vi "Create_Results_Row.vi"() -> (0 "row splitting":string[][](array[string]), 1 "Values to Keep in Dup rows":bool[](array[boolean]), 2 "Channel Values":string[](array[string]), 3 "Channel Names":string[](array[string]))   [LabVIEW 2015]
uses:
  Globals/Meas_global.vi
  Globals/Trav_pos_global.vi
  Globals/Dynamic_call_global.ph.vi
  Globals/Extra_Commands_Global.vi
  Globals/LDA_meas_global_1.vi
  Acquisition/PWA/PWAtasksGLOBAL.vi
panel:
  out "ScrollableArray":T1(array[cluster])
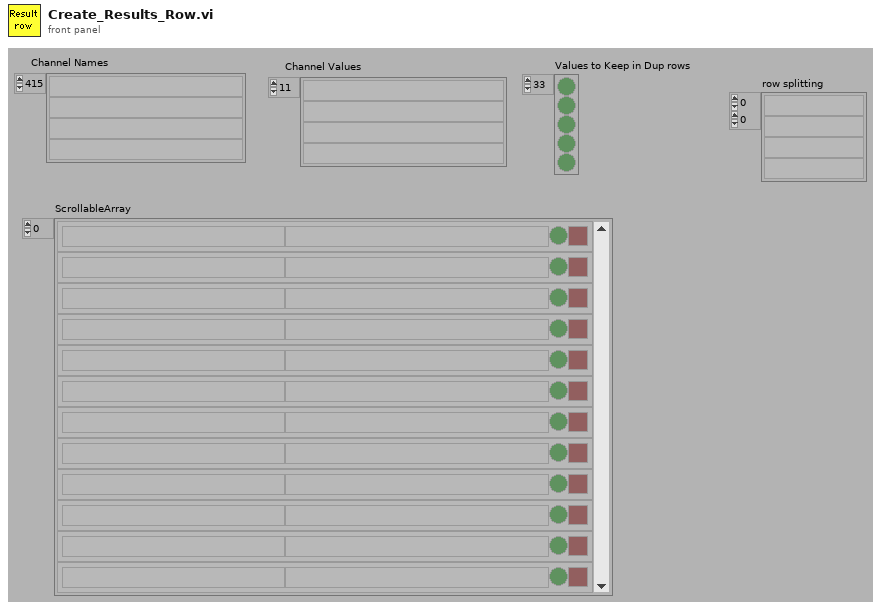
[diagram p1: front panel]
types:
  T1 = cluster{"Input Element":string, "name":string, bool, bool}[]
  T2 = typedef "Analysis_info_cluster.ctl" = cluster{"Colour":u32, "Inst type":T3, "Inst name":string, "Symbol":string, "Code name":string, "Extra Info":string, "Inst Array":T4, "Extra Titles":string[], "Extra Values":string[], "U":dbl, "u^2":dbl, "u^3":dbl, "u^4":dbl, "Skew_u":dbl, "Kurt_u":dbl, "Sd Error in Mean":dbl, "% u'/U":dbl, "X":dbl, "Y":dbl, "Z":dbl, "Timescale integral to 25%":dbl, "Sd Error in Variance":dbl, "Calib File":path, "Calib Constants":dbl[], "Output Position":bool, "Full Stats":bool, "Av Sampling Rate":dbl, "Av No of Samples":dbl, "Total Meas Time (s)":dbl, "ADAM Ch Name":string, "Max value":dbl, "Min value":dbl}
  T3 = typedef "Inst_type.ctl" = enum16{"Propeller anemometer", "Raw voltage", "Pressure Transducer", "Pitot-static tube", "Preston tube", "Hot wire", "Cross wire 1", "Cross wire 2", "Generic Linear", "Generic Polynomial", "Generic BackPoly", "Fast FID", "Thermocouple", "Cold wire", "Pulsed Wire", "LDA Vel", "LDA Tran time", "LDA Arr time", "Microphone"}
  T4 = typedef "Instrument_Array.ctl" = enum16{"PWA", "LDA", "Analogue"}
  T5 = typedef "Post_Process.ctl" = enum16{"Take New Data", "Post Process Raw Data File"}
  T6 = typedef "PWA_Data.ctl" = enum16{"No PWA Data", "One Ch PWA"}
  T7 = typedef "Correlation_cluster1.ctl" = cluster{"U inst":string, "uw":dbl, "u^2w":dbl, "uw^2":dbl, "uw/u'w'":dbl, "W inst":string, "uw^3":dbl, "u^3w":dbl, "u^2w^2":dbl, "Index U":i32, "Index W":i32}
  T8 = typedef "Traverse_cluster.ctl" = cluster{"Start X":sgl, "Start Y":sgl, "Start Z":sgl, "End X":sgl, "End Y":sgl, "End Z":sgl, "No. of pts.":i32, "Spacing":T9, "Filename":path, "Tunnel Speed":dbl, "Averaging time (min)":dbl, "Extra Commands":string, "Carrier_1 Q (l/min)":dbl, "Carrier_2 Q (l/min)":dbl, "Trace Gas Concentration (%)":dbl, "Specific Arguments":string, "Comments":string, "Row No":i32, "Row Type Selector":T10, "Completion time":string, "Row Duration (mins)":dbl, "No. of Valid pts.":i32, "Meas Setup File":string}
  T9 = typedef "Spacing.ctl" = enum16{"Linear", "Log", "Gauss", "Specified", "N/A"}
  T10 = typedef "Multi_run_mode.ctl" = enum16{"Move Traverse Only", "Set Tunnel Speed Only", "Set Source Only", "Set Measurement Conditions", "Single Measurement", "Vertical Profile", "Lateral Profile", "Longitudinal Profile", "Explore Volume", "Multi-Axis Profile", "Auto Calibrate", "Meas Fast FID Bkgnd", "Check Beam Power", "Scanning Valve Measurement", "Run VI Named:", "Set ADAM Ch", "Wait (minutes)", "Send Message", "Synchronize With:", "Fall Back to this Row", "Turn Off Row Repeating", "Blank Row", "Traverse 3D Volume"}
  T11 = cluster{"Input Element":string, "name":string, bool, bool}
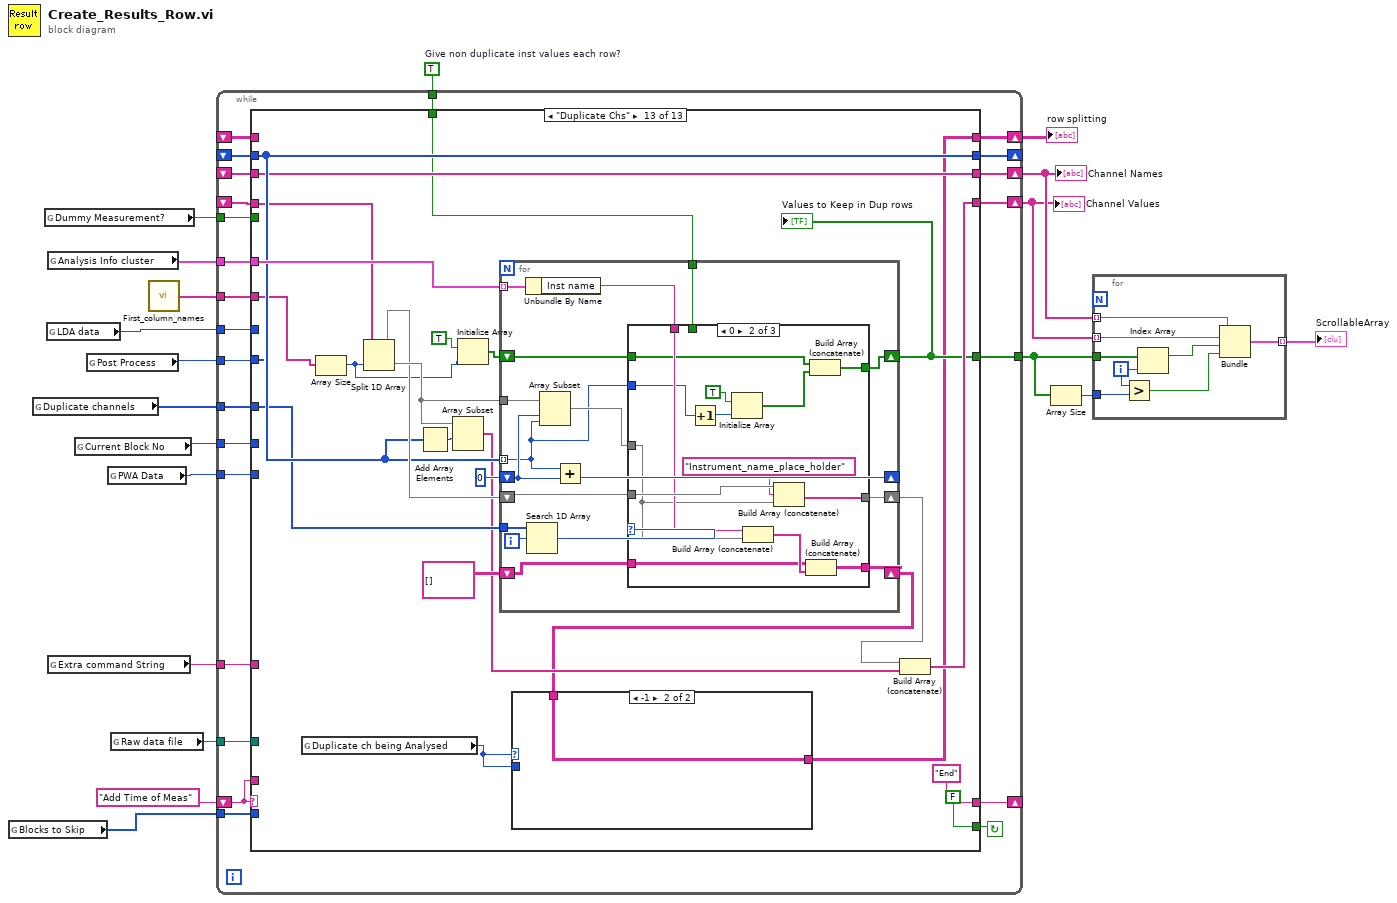
[diagram p0: block diagram]
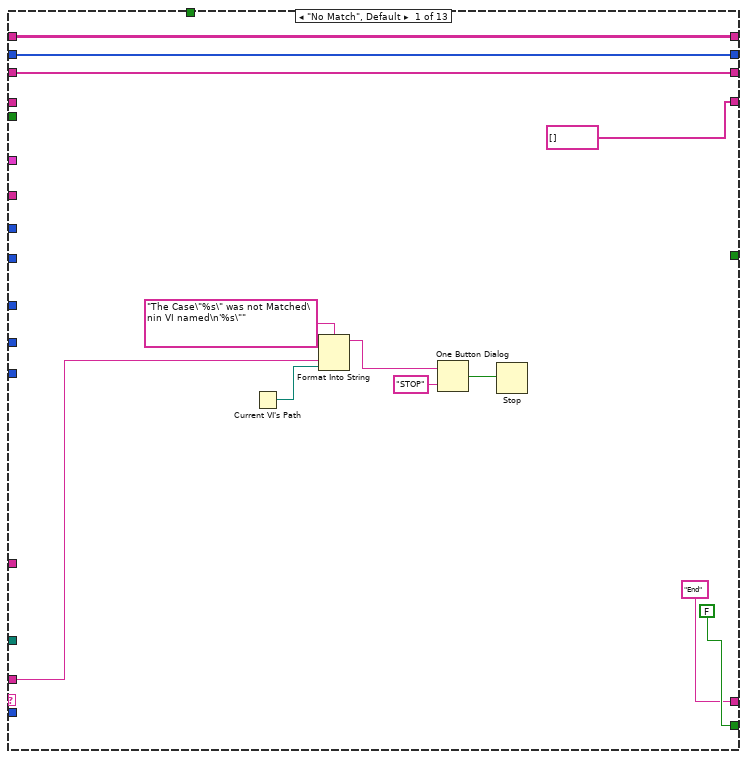
[diagram p2: hidden frame]
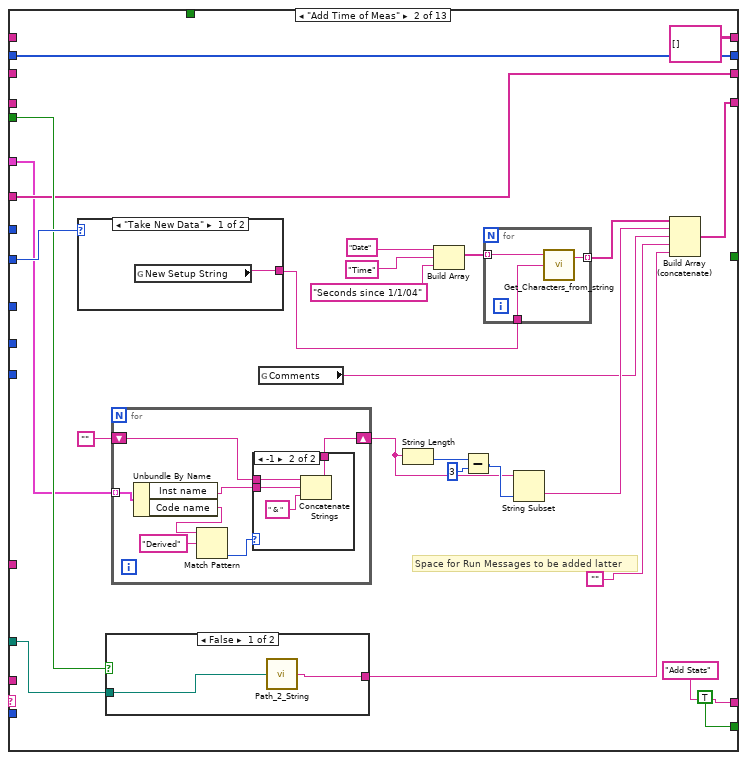
[diagram p3: hidden frame]
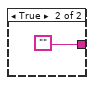
[diagram p4: hidden frame]
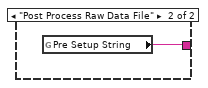
[diagram p6: hidden frame]
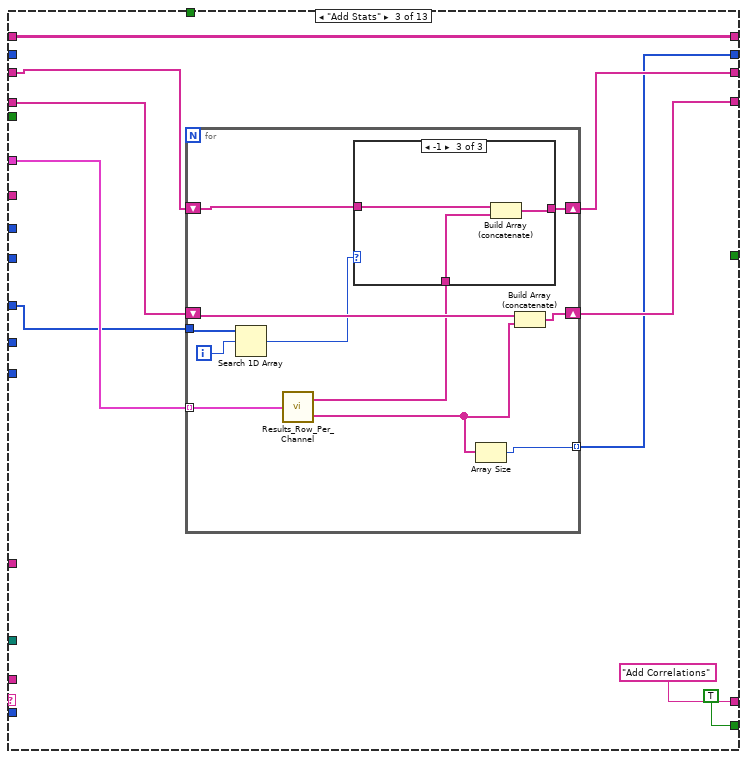
[diagram p7: hidden frame]
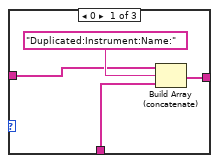
[diagram p8: hidden frame]
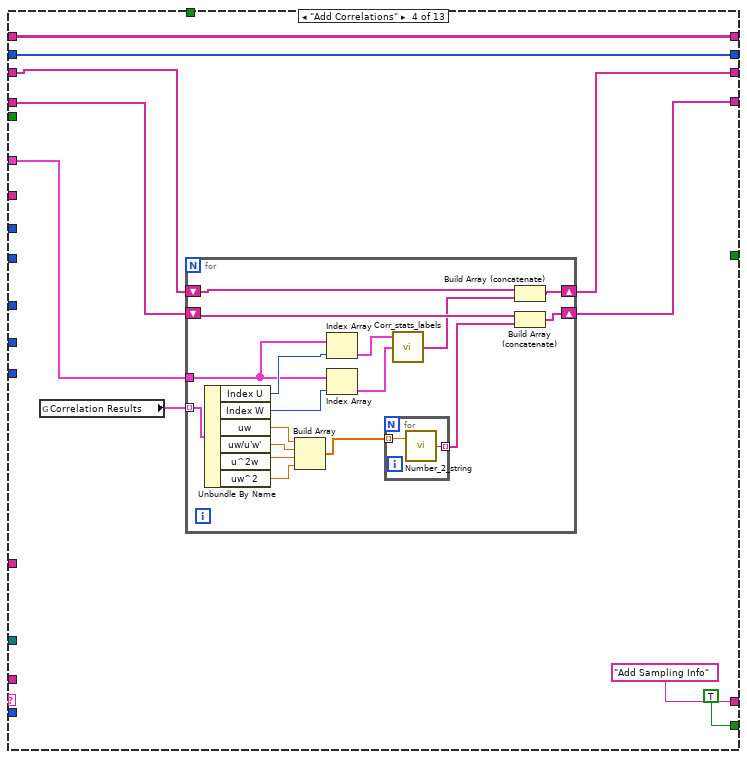
[diagram p10: hidden frame]
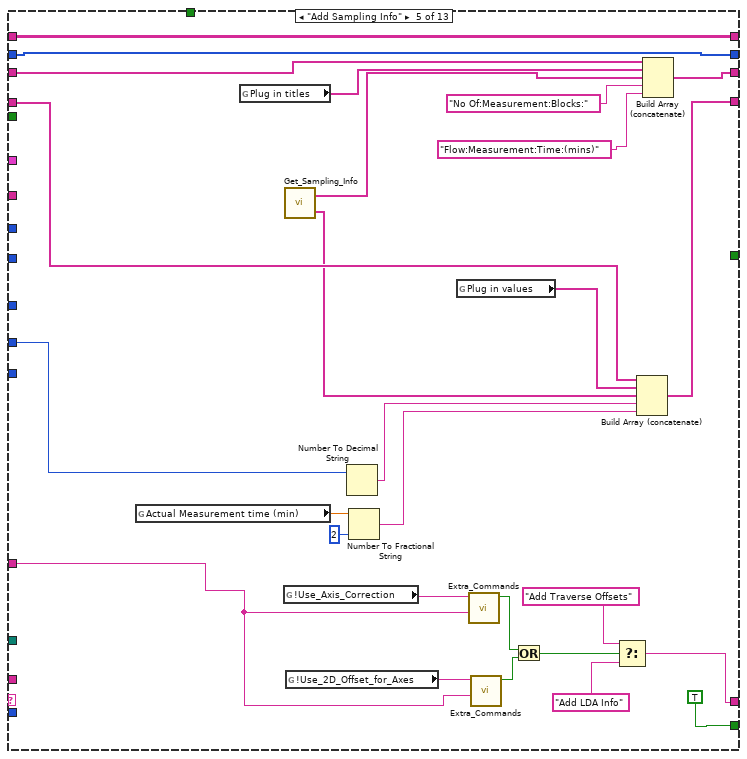
[diagram p11: hidden frame]
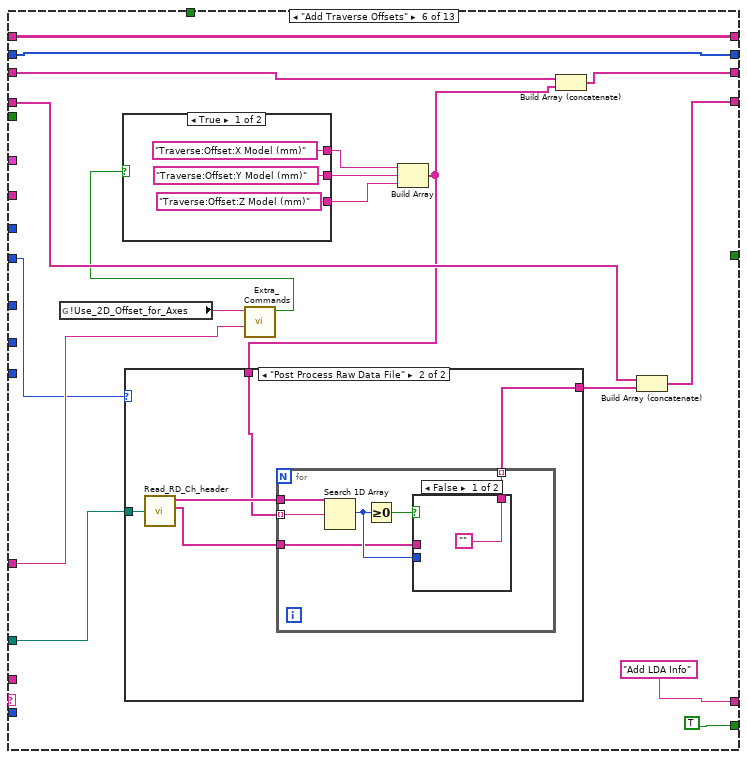
[diagram p12: hidden frame]
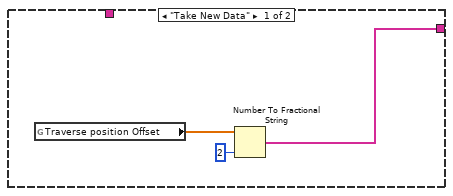
[diagram p13: hidden frame]
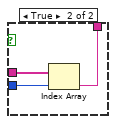
[diagram p14: hidden frame]
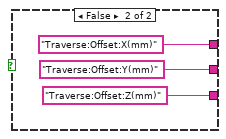
[diagram p15: hidden frame]
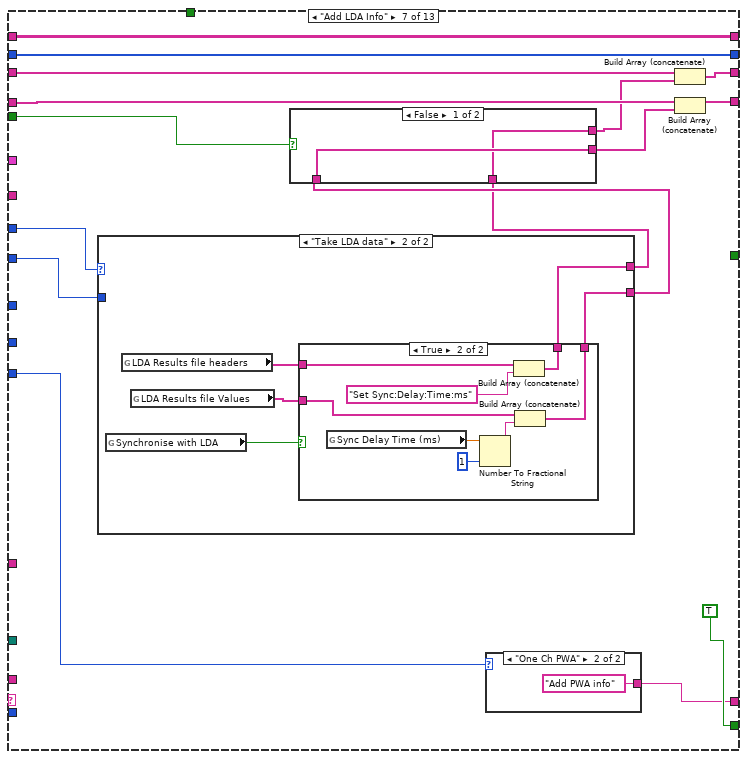
[diagram p16: hidden frame]
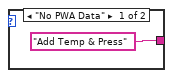
[diagram p17: hidden frame]
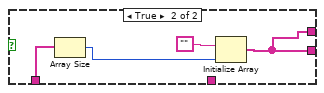
[diagram p18: hidden frame]
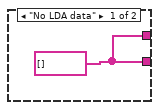
[diagram p19: hidden frame]
diagram:
  w1 = TRUE  # Give non duplicate inst values each row?
  n1 = global read "Meas_global.vi" "Blocks to Skip"() -> (w13:i32[])
  n2 = global read "Meas_global.vi" "Duplicate channels"() -> (w10:i32[])
  n3 = global read "Trav_pos_global.vi" "Dummy Measurement?"() -> (w15:bool)
  n4 = global read "Meas_global.vi" "LDA data"() -> (w19:enum16{"No LDA data", "Take LDA data"})
  n5 = global read "Meas_global.vi" "Analysis Info cluster"() -> (w17:T2[])
  n6 = global read "Meas_global.vi" "Extra command String"() -> (w7:string)
  n7 = global read "Meas_global.vi" "Current Block No"() -> (w18:i32)
  n8 = global read "Meas_global.vi" "Post Process"() -> (w16:T5)
  n9 = global read "Meas_global.vi" "PWA Data"() -> (w12:T6)
  n10 = global read "Meas_global.vi" "Raw data file"() -> (w11:path)
  n11 = call "First_column_names.vi"() -> ("Array"=w9:string[])
  n12 = while {
    shift-left: _ -> [w36]
    shift-right: [w37] -> w5
    shift-left: "Add Time of Meas" -> [w32]
    shift-right: [w38] -> _
    tunnel: w16 -> [w40]
    tunnel: w17 -> [w41]
    tunnel: w18 -> [w42]
    tunnel: w19 -> [w43]
    tunnel: w15 -> [w35]
    shift-right: [w34] -> w6
    shift-left: _ -> [w33]
    tunnel: w13 -> [w31]
    tunnel: w12 -> [w30]
    tunnel: w11 -> [w29]
    tunnel: w10 -> [w28]
    shift-right: [w27] -> _
    shift-left: _ -> [w26]
    tunnel: w9 -> [w25]
    shift-right: [w24] -> w8
    shift-left: _ -> [w23]
    tunnel: w7 -> [w22]
    tunnel: [w21] -> w4
    tunnel: w1 -> [w20]
    stop <- w39 continue-if-true
    n13 = case shown="\"Duplicate Chs\"" w32 {
      tunnel: w41 -> [_ w57 w106 w132 _ _ _ _ _ _ _ _ w518]
      tunnel: w43 -> [_ _ _ _ _ _ w241 _ _ _ _ _ _]
      tunnel: w42 -> [_ _ _ _ w181 _ _ w280 _ _ _ _ _]
      tunnel: w40 -> [_ w64 _ _ _ w190 w236 _ w354 _ w447 w489 _]
      tunnel: [FALSE ("Processing last block?") TRUE TRUE ("Processing last block?") TRUE ("Processing last block?") TRUE TRUE TRUE ("Processing last block?") TRUE ("Processing last block?") TRUE ("Processing last block?") TRUE ("Processing last block?") TRUE ("Processing last block?") w485 FALSE ("Processing last block?")] -> w39
      tunnel: ["End" "Add Stats" "Add Correlations" ("t") "Add Sampling Info" ("t") w161 "Add LDA Info" w230 "Add Temp & Press" "Replace Run Messages" "Add Plugins" "Add Original Results filename" "Duplicate Chs" "End" ("t")] -> w38
      tunnel: [string[] [] ("initialized array") w56 w107 w136 w180 w200 w242 w281 w362 w416 w442 w494 w511] -> w37
      tunnel: w36 -> [_ _ w108 w137 w177 w199 w243 w268 w349 w402 w448 w492 w515]
      tunnel: w32 -> [w50 _ _ _ _ _ _ _ _ _ _ _ _]
      tunnel: w35 -> [_ w63 _ _ _ _ w240 _ _ w410 _ _ _]
      tunnel: [w47 w59 w109 w138 w175 w187 w233 w271 w343 w408 w438 w482 w510] -> w34
      tunnel: w33 -> [w47 _ w110 w139 w176 w188 w234 w272 w348 w408 w440 w483 w510]
      tunnel: w31 -> [_ _ _ _ _ _ _ _ _ w404 _ _ _]
      tunnel: w30 -> [_ _ _ _ _ _ w231 _ _ _ _ _ _]
      tunnel: w29 -> [_ w61 _ _ _ w189 _ _ w353 _ _ _ _]
      tunnel: w28 -> [_ _ w103 _ _ _ _ _ _ _ _ w487 w514]
      tunnel: [w46 w60 w102 w131 w172 w198 w229 w270 w345 w401 w437 w488 w517] -> w27
      tunnel: w26 -> [w46 w60 _ w131 w172 w198 w229 w270 w345 w401 w437 w488 w517]
      tunnel: w25 -> [_ w59 _ _ _ _ _ _ _ _ _ _ w516]
      tunnel: [w45 string[][] [] w101 w130 w171 w197 w228 w269 w344 w400 w436 w484 w502] -> w24
      tunnel: w23 -> [w45 _ w101 w130 w171 w197 w228 w269 w344 w400 w436 w484 _]
      tunnel: w22 -> [_ _ _ _ w160 w192 _ _ _ _ _ _ _]
      tunnel: [_ _ _ _ _ _ _ _ _ _ _ _ w504] -> w21
      tunnel: w20 -> [_ _ _ _ _ _ _ _ _ _ _ _ w503]
      frame "No Match", Default {
        n14 = Current VI's Path() -> (path=w51:path)
        n15 = Format Into String(format string="The Case\"%s\" was not Matched\nin VI named\n'%s\"" ("Format String"), w50, w51) -> (resulting string=w54:string)  [unwired: 2 in, 1 out]
        n16 = One Button Dialog(message=w54, button name ("OK")="STOP") -> (true=w52:bool)
        n17 = Stop(stop? (T)=w52) -> ()
      }
      frame "Add Time of Meas" {
        # "Space for Run Messages to be added latter"
        n18 = case shown="\"Take New Data\"" w64 {
          tunnel: [w99 w100] -> w74
          frame "Take New Data" {
            n19 = global read "Meas_global.vi" "New Setup String"() -> (w99:string)
          }
          frame "Post Process Raw Data File" {
            n20 = global read "Meas_global.vi" "Pre Setup String"() -> (w100:string)
          }
        }
        n21 = case shown="False" w63 {
          tunnel: [w82 ""] -> w72
          tunnel: w61 -> [w81 _]
          frame False {
            n22 = call "Path_2_String.vi"("Real Path"=w81) -> ("Path String"=w82:string)
          }
          frame True {
          }
        }
        n23 = for {
          shift-right: [w89] -> w67
          shift-left: "" -> [w90]
          tunnel: w57 -> [w88] mode=indexing
          n24 = Unbundle By Name(w88) -> ("Inst name"=w87:string, "Code name"=w86:string)
          n25 = Match Pattern(string=w86, regular expression="Derived") -> (offset past match=w84:i32)  [unwired: 1 in, 3 out]
          n26 = case shown="-1" w84 {
            tunnel: w90 -> [w91 w95]
            tunnel: [w91 w94] -> w89
            tunnel: w87 -> [_ w92]
            frame 0, Default {
            }
            frame -1 {
              n27 = Concatenate Strings(w95, w92, " & ") -> (w94:string)
            }
          }
        }
        n28 = global read "Meas_global.vi" "Comments"() -> (w62:string)
        n29 = String Length(string=w67) -> (length=w70:i32)
        n30 = Build Array("Date", "Time", "Seconds since 1/1/04") -> (w76:string[])
        n31 = Subtract(x=w70, y=3) -> (x-y=w68:i32)
        n32 = for {
          tunnel: w76 -> [w98] mode=indexing
          tunnel: w74 -> [w97]
          tunnel: [w96] -> w75 mode=indexing
          n33 = call "Get_Characters_from_string.vi"("Input string"=w97, "Variable name"=w98) -> ("Value"=w96:string)  [unwired: 1 in, 1 out]
        }
        n34 = String Subset(string=w67, length (rest)=w68) -> (substring=w65:string)  [unwired: 1 out]
        n35 = Build Array (concatenate)(w75, w65, w62, "", w72) -> (w56:string[])
      }
      frame "Add Stats" {
        n36 = for {
          shift-right: [w118] -> w109
          shift-left: w110 -> [w120]
          shift-right: [w121] -> w107
          shift-left: w108 -> [w119]
          tunnel: w106 -> [w117] mode=indexing
          tunnel: [w114] -> w102 mode=indexing
          tunnel: w103 -> [w112]
          i -> [w113]
          n37 = Search 1D Array(1D array=w112, element=w113) -> (index of element=w111:i32)  [unwired: 1 out]
          n38 = call "Results_Row_Per_Channel.vi"("Analysis_info_cluster"=w117) -> ("Channel Names"=w116:string[], "Channel Values"=w115:string[])
          n39 = case shown="-1" w111 {
            tunnel: w120 -> [w124 w126 w129]
            tunnel: [w122 w126 w128] -> w118
            tunnel: w116 -> [w123 _ w127]
            frame 0 {
              n40 = Build Array (concatenate)(w124, "Duplicated:Instrument:Name:", w123) -> (w122:string[])
            }
            frame 1, Default {
            }
            frame -1 {
              n41 = Build Array (concatenate)(w129, w127) -> (w128:string[])
            }
          }
          n42 = Array Size(array=w115) -> (size(s)=w114:i32)
          n43 = Build Array (concatenate)(w119, w115) -> (w121:string[])
        }
      }
      frame "Add Correlations" {
        n44 = global read "Meas_global.vi" "Correlation Results"() -> (w133:T7[])
        n45 = for {
          shift-right: [w153] -> w138
          shift-left: w139 -> [w155]
          shift-right: [w156] -> w136
          shift-left: w137 -> [w154]
          tunnel: w133 -> [w152] mode=indexing
          tunnel: w132 -> [w149]
          n46 = Unbundle By Name(w152) -> ("Index U"=w151:i32, "Index W"=w150:i32, "uw"=w145:dbl, "uw/u'w'"=w144:dbl, "u^2w"=w143:dbl, "uw^2"=w142:dbl)
          n47 = Build Array(w145, w144, w143, w142) -> (w141:dbl[])
          n48 = Index Array(array=w149, index=w151) -> (element=w148:T2)
          n49 = Index Array(array=w149, index=w150) -> (element=w147:T2)
          n50 = for {
            tunnel: w141 -> [w158] mode=indexing
            tunnel: [w157] -> w140 mode=indexing
            n51 = call "Number_2_string.vi"("number"=w158) -> ("String"=w157:string)  [unwired: 1 in]
          }
          n52 = call "Corr_stats_labels.vi"("Inst 2 Units"=w147, "Inst 1 Units"=w148) -> ("Output"=w146:string[])  [unwired: 1 in]
          n53 = Build Array (concatenate)(w155, w146) -> (w153:string[])
          n54 = Build Array (concatenate)(w154, w140) -> (w156:string[])
        }
      }
      frame "Add Sampling Info" {
        n55 = global read "Meas_global.vi" "Actual Measurement time (min)"() -> (w182:dbl)
        n56 = global read "Dynamic_call_global.ph.vi" "Plug in titles"() -> (w174:string[])
        n57 = global read "Extra_Commands_Global.vi" "!Use_Axis_Correction"() -> (w164:string)
        n58 = call "Get_Sampling_Info.vi"() -> ("Channel Values"=w169:string[], "Channel Names"=w170:string[])  [unwired: 2 in]
        n59 = global read "Extra_Commands_Global.vi" "!Use_2D_Offset_for_Axes"() -> (w165:string)
        n60 = Number To Decimal String(number=w181) -> (decimal integer string=w179:string)  [unwired: 1 out]
        n61 = Number To Fractional String(number=w182, precision (6)=i16 2) -> (F-format string=w184:string)  [unwired: 2 out]
        n62 = global read "Dynamic_call_global.ph.vi" "Plug in values"() -> (w178:string[])
        n63 = call "Extra_Commands.vi"("String to Search"=w160, "Command"=w164) -> ("Command Found"=w166:bool)  [unwired: 1 in, 4 out]
        n64 = call "Extra_Commands.vi"("String to Search"=w160, "Command"=w165) -> ("Command Found"=w167:bool)  [unwired: 1 in, 4 out]
        n65 = Or(x=w166, y=w167) -> (x .or. y?=w159:bool)
        n66 = Select(t="Add Traverse Offsets", s=w159, f="Add LDA Info") -> (s? t:f=w161:string)
        n67 = Build Array (concatenate)(w177, w178, w169, w179, w184) -> (w180:string[])
        n68 = Build Array (concatenate)(w176, w174, w170, "No Of:Measurement:Blocks:", "Flow:Measurement:Time:(mins)") -> (w175:string[])
      }
      frame "Add Traverse Offsets" {
        n69 = global read "Extra_Commands_Global.vi" "!Use_2D_Offset_for_Axes"() -> (w193:string)
        n70 = call "Extra_Commands.vi"("String to Search"=w192, "Command"=w193) -> ("Command Found"=w191:bool)  [unwired: 1 in, 4 out]
        n71 = case shown="True" w191 {
          tunnel: ["Traverse:Offset:X Model (mm)" "Traverse:Offset:X(mm)"] -> w196
          tunnel: ["Traverse:Offset:Y Model (mm)" "Traverse:Offset:Y(mm)"] -> w195
          tunnel: ["Traverse:Offset:Z Model (mm)" "Traverse:Offset:Z(mm)"] -> w194
          frame True {
          }
          frame False {
          }
        }
        n72 = Build Array(w196, w195, w194) -> (w186:string[])
        n73 = case shown="\"Post Process Raw Data File\"" w190 {
          tunnel: [w206 w207] -> w201
          tunnel: w189 -> [_ w209]
          tunnel: w186 -> [_ w208]
          frame "Take New Data" {
            n74 = global read "Trav_pos_global.vi" "Traverse position Offset"() -> (w204:sgl[])
            n75 = Number To Fractional String(number=w204, precision (6)=i16 2) -> (F-format string=w206:string[])  [unwired: 2 out]
          }
          frame "Post Process Raw Data File" {
            n76 = call "Read_RD_Ch_header.vi"("Raw data file"=w209) -> ("Ch Name Out"=w211:string[], "Ch Values"=w210:string[])  [unwired: 2 out]
            n77 = for {
              tunnel: w211 -> [w217]
              tunnel: w210 -> [w214]
              tunnel: [w213] -> w207 mode=indexing
              tunnel: w208 -> [w212] mode=indexing
              n78 = Search 1D Array(1D array=w217, element=w212) -> (index of element=w215:i32)  [unwired: 1 out]
              n79 = Greater Or Equal To 0?(x=w215) -> (x >= 0?=w216:bool)
              n80 = case shown="False" w216 {
                tunnel: w215 -> [_ w221]
                tunnel: w214 -> [_ w220]
                tunnel: ["" w219] -> w213
                frame False {
                }
                frame True {
                  n81 = Index Array(array=w220, index=w221) -> (element=w219:string)
                }
              }
            }
          }
        }
        n82 = Build Array (concatenate)(w188, w186) -> (w187:string[])
        n83 = Build Array (concatenate)(w199, w201) -> (w200:string[])
      }
      frame "Add LDA Info" {
        n84 = case shown="\"Take LDA data\"" w241 {
          tunnel: w236 -> [_ _]
          tunnel: [w252 w253] -> w237
          tunnel: [w252 w255] -> w235
          frame "No LDA data" {
            w252 = string[] []
          }
          frame "Take LDA data" {
            n85 = global read "Meas_global.vi" "Synchronise with LDA"() -> (w257:bool)
            n86 = global read "LDA_meas_global_1.vi" "LDA Results file headers"() -> (w256:string[])
            n87 = global read "LDA_meas_global_1.vi" "LDA Results file Values"() -> (w254:string[])
            n88 = case shown="True" w257 {
              tunnel: w256 -> [w259 w265]
              tunnel: [w259 w263] -> w255
              tunnel: w254 -> [w258 w262]
              tunnel: [w258 w260] -> w253
              frame False {
              }
              frame True {
                n89 = global read "LDA_meas_global_1.vi" "Sync Delay Time (ms)"() -> (w266:dbl)
                n90 = Number To Fractional String(number=w266, precision (6)=i16 1) -> (F-format string=w261:string)  [unwired: 2 out]
                n91 = Build Array (concatenate)(w265, "Set Sync:Delay:Time:ms" ("Input Element")) -> (w263:string[])
                n92 = Build Array (concatenate)(w262, w261) -> (w260:string[])
              }
            }
          }
        }
        n93 = case shown="False" w240 {
          tunnel: [w247 w248] -> w239
          tunnel: w237 -> [w247 w251]
          tunnel: [w246 w248] -> w232
          tunnel: w235 -> [w246 _]
          frame False {
          }
          frame True {
            n94 = Array Size(array=w251) -> (size(s)=w250:i32)
            n95 = Initialize Array("", w250) -> (w248:string[])
          }
        }
        n96 = case shown="\"One Ch PWA\"" w231 {
          tunnel: ["Add Temp & Press" "Add PWA info"] -> w230
          frame "No PWA Data" {
          }
          frame "One Ch PWA" {
          }
        }
        n97 = Build Array (concatenate)(w234, w232) -> (w233:string[])
        n98 = Build Array (concatenate)(w243, w239) -> (w242:string[])
      }
      frame "Add PWA info" {
        n99 = stacked-sequence {
          tunnel: w280 -> [w309 _ _]
          tunnel: [w304 _ _] -> w279
          tunnel: [w299 _ _] -> w278
          tunnel: [w298 _ _] -> w277
          tunnel: [_ w312 _] -> w276
          tunnel: [_ w311 _] -> w275
          tunnel: [w292 _ _] -> w274
          tunnel: [w284 _ _] -> w273
          tunnel: w272 -> [_ _ w331]
          tunnel: [_ _ w330] -> w271
          frame #0 {
            n100 = global read "PWAtasksGLOBAL.vi" "PWA No. of Samples"() -> (w310:i32)
            n101 = global read "PWAtasksGLOBAL.vi" "PWA No of  TOF Timeouts"() -> (w289:i32)
            n102 = global read "PWAtasksGLOBAL.vi" "PWA No of  TOF Below Min"() -> (w290:i32)
            n103 = Multiply(x=w310, y=w309) -> (x*y=w291:i32)
            n104 = global read "PWAtasksGLOBAL.vi" "PWA Setup summary"() -> (w298:string)
            n105 = global read "PWAtasksGLOBAL.vi" "PWA Seconds per clock pulse"() -> (w296:dbl)
            n106 = Compound Arithmetic op=ADD(w291, invert w290, invert w289) -> (w287:i32)
            n107 = global read "PWAtasksGLOBAL.vi" "PWA No of Reverse samples"() -> (w288:i32)
            n108 = global read "PWAtasksGLOBAL.vi" "Minimum TOF Index"() -> (w297:i16)
            n109 = Divide(x=w289, y=w291) -> (x/y=w308:dbl)
            n110 = Divide(x=w290, y=w291) -> (x/y=w300:dbl)
            n111 = Multiply(x=w308, y=100.0) -> (x*y=w305:dbl)
            n112 = Multiply(x=w300, y=100.0) -> (x*y=w303:dbl)
            n113 = Number To Fractional String(number=w305, precision (6)=i16 2) -> (F-format string=w304:string)  [unwired: 2 out]
            n114 = Number To Fractional String(number=w303, precision (6)=i16 2) -> (F-format string=w299:string)  [unwired: 2 out]
            n115 = Multiply(x=w296, y=w297) -> (x*y=w295:dbl)
            n116 = Divide(x=w288, y=w287) -> (x/y=w285:dbl)
            n117 = Multiply(x=w295, y=1000000.0) -> (x*y=w293:dbl)
            n118 = Number To Fractional String(number=w285, precision (6)=i16 6) -> (F-format string=w284:string)  [unwired: 2 out]
            n119 = Number To Decimal String(number=w293) -> (decimal integer string=w292:string)  [unwired: 1 out]
          }
          frame #1 {
            w325 = 4095
            w321 = 4095
            n120 = global read "PWAtasksGLOBAL.vi" "Minimum TOF Index"() -> (w320:i16)
            n121 = global read "PWAtasksGLOBAL.vi" "PWA Lookup Table"() -> (w324:dbl[])
            n122 = Negate(x=w321) -> (-x=w323:i32)
            n123 = Negate(x=w320) -> (-x=w322:i16)
            n124 = Add(x=w321, y=w325) -> (x+y=w326:i32)
            n125 = Add(x=w320, y=w325) -> (x+y=w327:i32)
            n126 = Add(x=w322, y=w325) -> (x+y=w329:i32)
            n127 = Add(x=w323, y=w325) -> (x+y=w328:i32)
            n128 = Index Array(array=w324, index=w326) -> (element=w319:dbl)
            n129 = Index Array(array=w324, index=w327) -> (element=w318:dbl)
            n130 = Index Array(array=w324, index=w328) -> (element=w315:dbl)
            n131 = Index Array(array=w324, index=w329) -> (element=w313:dbl)
            n132 = global read "PWAtasksGLOBAL.vi" "PWA Symbol"() -> (w314:string)
            n133 = Format Into String(format string="%.3f<%s<%.2f", w319, w314, w318) -> (resulting string=w312:string)  [unwired: 2 in, 1 out]
            n134 = Format Into String(format string=" %.3f<%s<%.2f", w315, w314, w313) -> (resulting string=w311:string)  [unwired: 2 in, 1 out]
          }
          frame #2 {
            n135 = global read "PWAtasksGLOBAL.vi" "PWA Symbol"() -> (w334:string)
            n136 = Format Into String(format string="PWA:Positive Wire:%s Limits:", w334) -> (resulting string=w338:string)  [unwired: 2 in, 1 out]
            n137 = Format Into String(format string="PWA:Negative Wire:%s Limits:", w334) -> (resulting string=w339:string)  [unwired: 2 in, 1 out]
            n138 = Build Array (concatenate)(w331, "PWA:Minimum:TOF:Micro-Sec", "PWA:% of TOF:Timeouts:", "PWA:% of TOF:Below Min:", "PWA:Setup:Info:", "PWA:Reverse:Flow Factor:0-1", w338, w339) -> (w330:string[])
          }
        }
        n139 = Build Array (concatenate)(w268, w274, w279, w278, w277, w273, w276, w275) -> (w281:string[])
      }
      frame "Add Temp & Press" {
        w342 = string[] ["Multi Run:Command:Filename", "Multi Run:Start Time:", "Multi Run:Duration in:Minutes", "Multi Run:Row:Type", "Multi Run:Row:Number", "Multi Run:Extra:Command"] ("appended array")
        n140 = case shown="\"Post Process Raw Data File\"" w354 {
          tunnel: [w374 w386] -> w355
          tunnel: w353 -> [_ w389]
          tunnel: w342 -> [_ w385]
          frame "Take New Data" {
            n141 = global read "Meas_global.vi" "Start Time of experiment"() -> (w368:dbl)
            n142 = global read "Trav_pos_global.vi" "Current Row"() -> (w380:T8)
            n143 = Get Date/Time In Seconds() -> (seconds since 1Jan1904=w370:timestamp)
            n144 = global read "Trav_pos_global.vi" "Top level setup filename"() -> (w373:path)
            n145 = To Double Precision Float(number=w370) -> (double precision float=w369:dbl)
            n146 = Unbundle By Name(w380) -> ("Row Type Selector"=w379:T10, "Row No"=w376:i32, "Extra Commands"=w371:string)
            n147 = Subtract(x=w369, y=w368) -> (x-y=w367:dbl)
            n148 = Divide(x=w367, y=60.0) -> (x/y=w365:dbl)
            n149 = call "Sec_to_date_filename.vi"("seconds"=w368) -> ("Day"=w383:string, "Time"=w384:string)  [unwired: 2 out]
            n150 = Strip Path(path=w373) -> (name=w372:string)  [unwired: 1 out]
            n151 = Number To Fractional String(number=w365, precision (6)=i16 1) -> (F-format string=w363:string)  [unwired: 2 in]
            n152 = Format Into String(format string="%s", w379) -> (resulting string=w377:string)  [unwired: 2 in, 1 out]
            n153 = Number To Decimal String(number=w376) -> (decimal integer string=w375:string)  [unwired: 1 in]
            n154 = Format Into String(format string="%s on %s", w384, w383) -> (resulting string=w381:string)  [unwired: 2 in, 1 out]
            n155 = Build Array(w372, w381, w363, w377, w375, w371) -> (w374:string[])
          }
          frame "Post Process Raw Data File" {
            n156 = call "Read_RD_Ch_header.vi"("Raw data file"=w389) -> ("Ch Name Out"=w388:string[], "Ch Values"=w387:string[])  [unwired: 2 out]
            n157 = for {
              tunnel: w388 -> [w395]
              tunnel: w387 -> [w392]
              tunnel: [w391] -> w386 mode=indexing
              tunnel: w385 -> [w390] mode=indexing
              n158 = Search 1D Array(1D array=w395, element=w390) -> (index of element=w393:i32)  [unwired: 1 out]
              n159 = Greater Or Equal To 0?(x=w393) -> (x >= 0?=w394:bool)
              n160 = case shown="False" w394 {
                tunnel: w393 -> [_ w399]
                tunnel: w392 -> [_ w398]
                tunnel: ["" w397] -> w391
                frame False {
                }
                frame True {
                  n161 = Index Array(array=w398, index=w399) -> (element=w397:string)
                }
              }
            }
          }
        }
        n162 = global read "Meas_global.vi" "Abs Press (mbar)"() -> (w360:dbl)
        n163 = global read "Meas_global.vi" "Temp"() -> (w356:dbl)
        n164 = Number To Fractional String(number=w360, precision (6)=i16 2) -> (F-format string=w361:string)  [unwired: 2 out]
        n165 = Number To Fractional String(number=w356, precision (6)=i16 1) -> (F-format string=w358:string)  [unwired: 2 out]
        n166 = Build Array (concatenate)(w358, w361, w355) -> (w350:string[])
        n167 = Build Array (concatenate)(w348, "Reference:Temperature:Used for Corrections", "Atmos:Pressure:Used for Corrections", w342) -> (w343:string[])
        n168 = Build Array (concatenate)(w349, w350) -> (w362:string[])
      }
      frame "Replace Run Messages" {
        n169 = Array Size(array=w404) -> (size(s)=w405:i32)
        n170 = global read "Meas_global.vi" "BSA data rate string"() -> (w418:string)
        n171 = global read "Meas_global.vi" "Over/Under string"() -> (w420:string)
        n172 = Equal To 0?(x=w405) -> (x = 0?=w403:bool)
        n173 = global read "Meas_global.vi" "Extra Comments"() -> (w419:string)
        n174 = Concatenate Strings(w418, w420, w419) -> (w417:string)
        n175 = call "Remove_unprintable_Char.vi"("Input String"=w417) -> ("Output String"=w407:string)
        n176 = case shown="False" w403 {
          tunnel: w404 -> [w426 _]
          tunnel: w407 -> [w422 w431]
          tunnel: [w421 w431] -> w406
          frame False {
            n177 = for {
              shift-right: [w428] -> w424
              shift-left: "Blocks " -> [w430]
              tunnel: w426 -> [w429] mode=indexing
              n178 = Format Into String(format string="%d; ", initial string=w430, w429) -> (resulting string=w428:string)  [unwired: 1 in, 1 out]
            }
            n179 = Concatenate Strings(w422, w424, "have been skipped. " ("string")) -> (w421:string)
          }
          frame True {
          }
        }
        n180 = case shown="False" w410 {
          tunnel: [w432 "Dummy Measurement"] -> w409
          tunnel: w406 -> [w432 _]
          frame False {
          }
          frame True {
          }
        }
        n181 = call "First_column_names.vi"() -> ("Array"=w413:string[])
        n182 = Search 1D Array(1D array=w413, element="Run:Messages::") -> (index of element=w412:i32)  [unwired: 1 out]
        n183 = Replace Array Subset(array=w402, new element=w409, index=w412) -> (w416:string[])
      }
      frame "Add Plugins" {
        n184 = case shown="\"Take New Data\"" w447 {
          tunnel: ["Take New Data" "Post Process"] -> w446
          frame "Take New Data" {
          }
          frame "Post Process Raw Data File" {
          }
        }
        n185 = global read "Meas_global.vi" "Acquisition vi to Run"() -> (w434:string)
        n186 = Build Array (concatenate)(w440, "Prog Post:Process:Mode" ("Input Element"), "Acquisition:PlugIn:Used" ("Input Element")) -> (w439:string[])
        n187 = Build Array (concatenate)(w448, w446, w434) -> (w443:string[])
        n188 = for {
          N: 3 -> [_]
          shift-right: [w455] -> w442
          shift-left: w443 -> [w456]
          shift-right: [w451] -> w438
          shift-left: w439 -> [w452]
          i -> [w459]
          n189 = case shown="0, Default" w459 {
            tunnel: [w470 w472 w474] -> w453
            tunnel: ["Initial:PlugIns:Used" ("Input Element") "Per Block:PlugIns:Used" ("Input Element") "Final:PlugIns:Used" ("Input Element")] -> w450
            frame 0, Default {
              n190 = global read "Dynamic_call_global.ph.vi" "Initial Plug Ins"() -> (w470:string[])
            }
            frame 1 {
              n191 = global read "Dynamic_call_global.ph.vi" "Per Block Plug Ins"() -> (w472:string[])
            }
            frame 2 {
              n192 = global read "Dynamic_call_global.ph.vi" "Final Plug Ins"() -> (w474:string[])
            }
          }
          n193 = Array Size(array=w453) -> (size(s)=w458:i32)
          n194 = for {
            tunnel: w453 -> [w475] mode=indexing
            shift-right: [w476] -> w454
            shift-left: "" -> [w478]
            n195 = Concatenate Strings(w478, w475, ";" ("string")) -> (w476:string)
          }
          n196 = Greater Than 0?(x=w458) -> (x > 0?=w457:bool)
          n197 = case shown="True" w457 {
            tunnel: w456 -> [w462 w468]
            tunnel: [w462 w467] -> w455
            tunnel: w454 -> [_ w466]
            tunnel: w452 -> [w461 w465]
            tunnel: [w461 w464] -> w451
            tunnel: w450 -> [_ w463]
            frame False {
            }
            frame True {
              n198 = Build Array (concatenate)(w468, w466) -> (w467:string[])
              n199 = Build Array (concatenate)(w465, w463) -> (w464:string[])
            }
          }
        }
      }
      frame "Add Original Results filename" {
        n200 = case shown="\"Take New Data\"" w489 {
          tunnel: [w495 w499] -> w491
          frame "Post Process Raw Data File" {
            n201 = global read "Meas_global.vi" "Pre Setup String"() -> (w498:string)
            n202 = call "Get_Characters_from_string.vi"("Input string"=w498, "Variable name"="Results filename") -> ("Value"=w496:string)  [unwired: 1 in, 1 out]
            n203 = call "String_to_Pathname.vi"("Input String"=w496) -> ("path"=w495:path)
          }
          frame "Take New Data" {
            n204 = global read "Meas_global.vi" "Results file"() -> (w499:path)
          }
        }
        n205 = Array Size(array=w487) -> (size(s)=w486:i32)
        n206 = Not Equal To 0?(x=w486) -> (x != 0?=w485:bool)
        n207 = Strip Path(path=w491) -> (name=w490:string)  [unwired: 1 out]
        n208 = Build Array (concatenate)(w483, "Original:Results:Filename") -> (w482:string[])
        n209 = Build Array (concatenate)(w492, w490) -> (w494:string[])
      }
      frame "Duplicate Chs" {
        n210 = global read "Meas_global.vi" "Duplicate ch being Analysed"() -> (w500:i32)
        n211 = Array Size(array=w516) -> (size(s)=w506:i32)
        n212 = Split 1D Array(array=w515, index=w506) -> (first subarray=w520:string[], second subarray=w522:string[])
        n213 = Add Array Elements(numeric array=w517) -> (sum=w521:i32)
        n214 = Array Subset(array=w522, index=w521) -> (w512:string[])  [unwired: 1 in]
        n215 = Initialize Array(TRUE, w506) -> (w505:bool[])
        n216 = for {
          shift-right: [w543] -> w513
          shift-left: w520 -> [w544]
          tunnel: w517 -> [w532] mode=indexing
          tunnel: w522 -> [w545]
          shift-right: [w542] -> _
          shift-left: 0 -> [w541]
          tunnel: w514 -> [w539]
          shift-right: [w537] -> w501
          shift-left: string[][] [] -> [w536]
          tunnel: w518 -> [w533] mode=indexing
          shift-right: [w530] -> w504
          shift-left: w505 -> [w531]
          tunnel: w503 -> [w529]
          i -> [w535]
          n217 = Unbundle By Name(w533) -> ("Inst name"=w534:string)
          n218 = Search 1D Array(1D array=w539, element=w535) -> (index of element=w538:i32)  [unwired: 1 out]
          n219 = Array Subset(array=w545, index=w541, length=w532) -> (w540:string[])
          n220 = Add(x=w532, y=w541) -> (x+y=w542:i32)
          n221 = case shown="0" w538 {
            tunnel: w544 -> [w554 w567 w570]
            tunnel: [w553 w568 w570] -> w543
            tunnel: w540 -> [w552 w564 w574]
            tunnel: w534 -> [_ w565 w575]
            tunnel: [w551 w562 w572] -> w537
            tunnel: w536 -> [w551 w561 w571]
            tunnel: w532 -> [w550 w556 _]
            tunnel: w531 -> [w548 w559 w569]
            tunnel: [w547 w558 w569] -> w530
            tunnel: w529 -> [w546 _ _]
            frame -1 {
              n222 = Initialize Array(w546, w550) -> (w549:bool[])
              n223 = Build Array (concatenate)(w554, w552) -> (w553:string[])
              n224 = Build Array (concatenate)(w548, w549) -> (w547:bool[])
            }
            frame 0 {
              n225 = Increment(x=w556) -> (x+1=w555:i32)
              n226 = Initialize Array(TRUE, w555) -> (w557:bool[])
              n227 = Build Array (concatenate)(w565, w564) -> (w563:string[])
              n228 = Build Array (concatenate)(w567, "Instrument_name_place_holder", w564) -> (w568:string[])
              n229 = Build Array (concatenate)(w561, w563) -> (w562:string[][])
              n230 = Build Array (concatenate)(w559, w557) -> (w558:bool[])
            }
            frame 1, Default {
              n231 = Build Array (concatenate)(w575, w574) -> (w573:string[])
              n232 = Build Array (concatenate)(w571, w573) -> (w572:string[][])
            }
          }
        }
        "Values to Keep in Dup rows" <- w504
        n233 = case shown="-1" w500 {
          tunnel: [w524 w528] -> w502
          tunnel: w501 -> [w527 w528]
          tunnel: w500 -> [w526 _]
          frame Default {
            n234 = Index Array(array=w527, index (row)=w526) -> (element=w525:string[])  [unwired: 1 in]
            n235 = Build Array(w525) -> (w524:string[][])
          }
          frame -1 {
          }
        }
        n236 = Build Array (concatenate)(w513, w512) -> (w511:string[])
      }
    }
  }
  "Channel Values" <- w5
  "Channel Names" <- w6
  "row splitting" <- w8
  n237 = Array Size(array=w4) -> (size(s)=w3:i32)
  n238 = for {
    tunnel: w6 -> [w583] mode=indexing
    tunnel: w5 -> [w582] mode=indexing
    tunnel: w4 -> [w581]
    tunnel: [w580] -> w2 mode=indexing
    tunnel: w3 -> [w577]
    i -> [w578]
    n239 = Greater?(x=w578, y=w577) -> (0:w576:bool)
    n240 = Index Array(array=w581, index=w578) -> (element=w579:bool)
    n241 = Bundle("Input Element"=w583, "name"=w582, w579, w576) -> (w580:T11)  [unwired: 1 in]
  }
  "ScrollableArray" <- w2
